vi "Process Packet.vi"(8 "error in (no error)":errorcluster, 10 "Incoming Packet":refnum<class "ControlPacket.lvclass">, 11 "Session in":refnum<class "Session.lvclass">) -> (0 "error out":errorcluster, 3 "Session out":refnum<class "Session.lvclass">)   [LabVIEW 2013, in "MQTT Base.lvlib" / "Session.lvclass"]
uses:
  Session.lvclass
  <vilib>/LabVIEW Open Source Project/MQTT Control Packets/Control Packets/ControlPacket/ControlPacket.lvclass
  Base Class/Request -- cluster.ctl
  Base Class/Response -- cluster.ctl
  Session.lvclass/Session.ctl
  <vilib>/LabVIEW Open Source Project/MQTT Control Packets/Control Packets/ControlPacket/ControlPacket.lvclass/ControlPacket.ctl
  Read SessionState.vi
  Base Class/MQTT_Base.lvclass
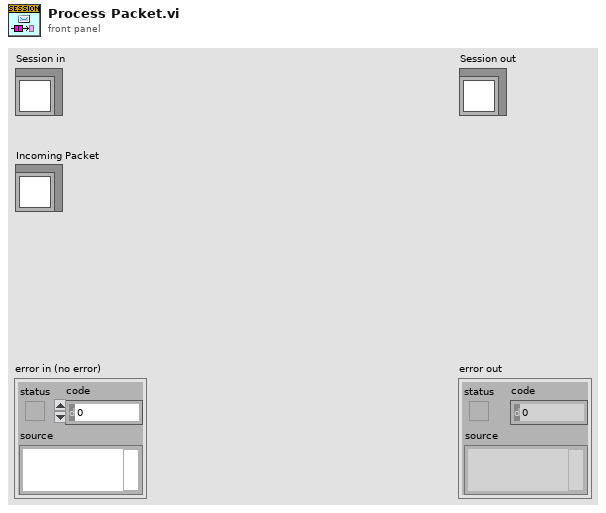
[diagram p1: front panel]
types:
  T1 = typedef "MQTT Base.lvlib/MQTT_Base.lvclass/Request -- cluster.ctl" = cluster{"Packet":refnum<class "ControlPacket.lvclass">, "SessionMailbox":refnum<queue>}
  T2 = typedef "MQTT Base.lvlib/MQTT_Base.lvclass/Response -- cluster.ctl" = cluster{"Packet":refnum<class "ControlPacket.lvclass">, "Protocol Error":errorcluster, "disconnect session":bool, "[ACK]":refnum<notifier>[]}
  T3 = typedef "MQTT Base.lvlib/Session.lvclass/Pending ACKs -- cluster.ctl" = cluster{"Message":refnum<class "ControlPacket.lvclass">, "[ACK]":refnum<notifier>[], "Packet Identifier":u16}
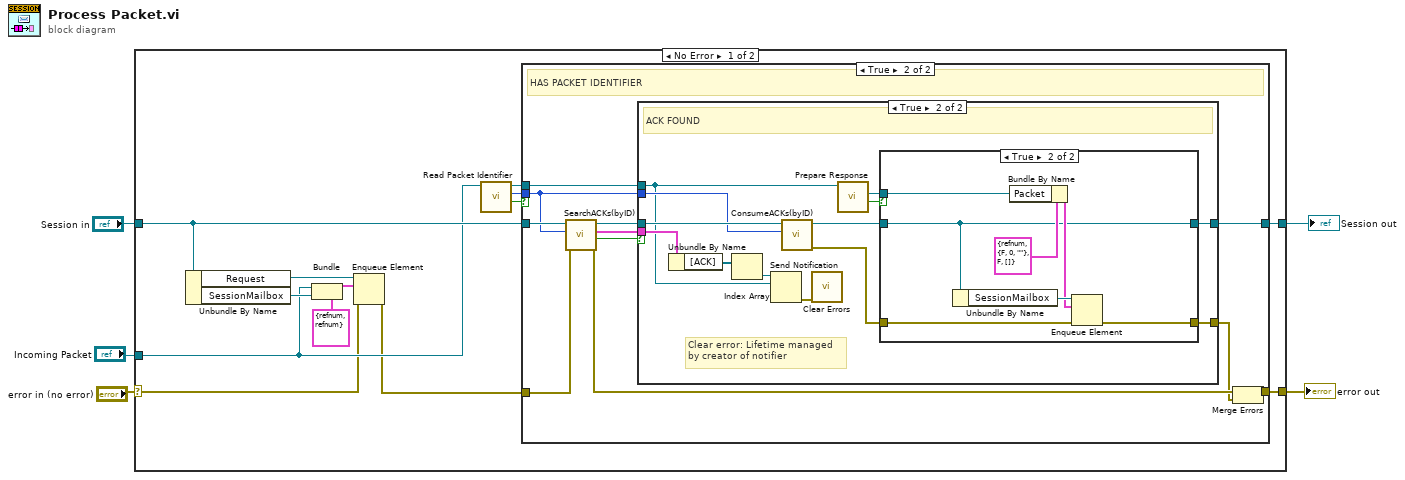
[diagram p0: block diagram]
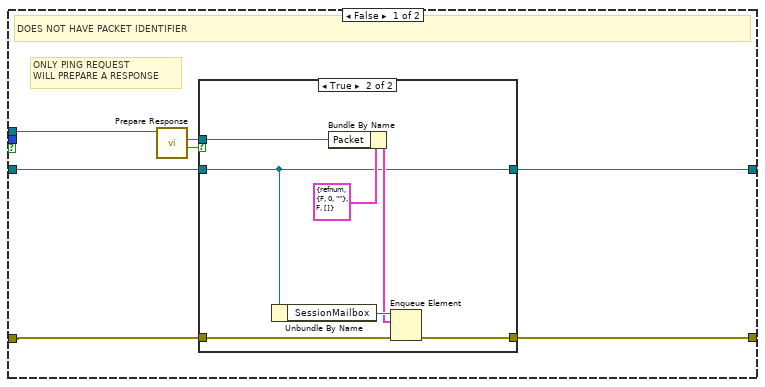
[diagram p2: hidden frame]
diagram:
  n1 = case shown="No Error" "error in (no error)" {
    selector: "error in (no error)" -> [w8 w70]
    tunnel: [w18 w70] -> w1
    tunnel: [w15 w69] -> w2
    tunnel: "Session in" -> [w10 w69]
    tunnel: "Incoming Packet" -> [w9 _]
    frame No Error {
      n2 = Unbundle By Name(w10) -> ("Request"=w11:refnum<queue>, "SessionMailbox"=w12:refnum<queue>)
      n3 = Bundle(cluster=T1 {"Packet"=refnum, "SessionMailbox"=refnum} ("Request"), "Packet"=w9, "SessionMailbox"=w12) -> (w13:T1)
      n4 = Enqueue Element(queue=w11, element=w13, error in (no error)=w8) -> (error out=w7:errorcluster)  [unwired: 1 in, 2 out]
      n5 = call <vilib>:"Read Packet Identifier.vi"("ControlPacket in"=w9) -> ("Has Packet Identifier"=w6:bool, "Packet Identifier"=w17:u16, "ControlPacket out"=w16:refnum<class "ControlPacket.lvclass">)  [unwired: 8 in]
      n6 = case shown="True" w6 {
        tunnel: [w19 w42] -> w18
        tunnel: w17 -> [_ w35]
        tunnel: w16 -> [w21 w41]
        tunnel: [w23 w39] -> w15
        tunnel: w10 -> [w24 w37]
        tunnel: w7 -> [w20 w36]
        frame False {
          # "ONLY PING REQUEST\nWILL PREPARE A RESPONSE"
          # "DOES NOT HAVE PACKET IDENTIFIER"
          n7 = call-dynamic "Prepare Response.vi"("ControlPacket in"=w21) -> ("response prepared?"=w22:bool, "ControlPacket response"=w25:refnum<class "ControlPacket.lvclass">)  [unwired: 7 in, 2 out]
          n8 = case shown="True" w22 {
            tunnel: w24 -> [w27 w29]
            tunnel: [w26 w31] -> w19
            tunnel: [w27 w29] -> w23
            tunnel: w25 -> [_ w30]
            tunnel: w20 -> [w26 w28]
            frame False {
            }
            frame True {
              n9 = Unbundle By Name(w29) -> ("SessionMailbox"=w34:refnum<queue>)
              n10 = Bundle By Name(cluster=T2 {"Packet"=refnum, "Protocol Error"={"status"=FALSE, "code"=0, "source"=""}, "disconnect session"=FALSE, "[ACK]"=[]} ("element"), "Packet"=w30) -> (w32:T2)
              n11 = Enqueue Element(queue=w34, element=w32, error in (no error)=w28) -> (error out=w31:errorcluster)  [unwired: 1 in, 2 out]
            }
          }
        }
        frame True {
          # "HAS PACKET IDENTIFIER"
          n12 = call "SearchACKs(byID).vi"("error in (no error)"=w36, "Packet Identifier"=w35, "Session in"=w37) -> ("error out"=w40:errorcluster, "found?"=w45:bool, "Pending ACK"=w44:T3, "Session out"=w43:refnum<class "Session.lvclass">)  [unwired: 5 in]
          n13 = case shown="True" w45 {
            tunnel: w44 -> [_ w56]
            tunnel: w43 -> [w46 w55]
            tunnel: [w46 w54] -> w39
            tunnel: w41 -> [_ w47]
            tunnel: [_ w53] -> w38
            tunnel: w35 -> [_ w48]
            frame False {
            }
            frame True {
              # "Clear error: Lifetime managed\nby creator of notifier"
              # "ACK FOUND"
              n14 = Unbundle By Name(w56) -> ("[ACK]"=w59:refnum<notifier>[])
              n15 = Index Array(array=w59) -> (element=w58:refnum<notifier>)  [unwired: 1 in]
              n16 = Send Notification(notification=w47, notifier=w58) -> (error out=w57:errorcluster)  [unwired: 1 in, 1 out]
              n17 = call "ConsumeACKs(byID).vi"("Packet Identifier"=w48, "Session in"=w55) -> ("error out"=w49:errorcluster, "Session out"=w50:refnum<class "Session.lvclass">)  [unwired: 8 in]
              n18 = call <vilib>:"Clear Errors.vi"("error in (no error)"=w57) -> ()  [unwired: 6 in, 1 out]
              n19 = call-dynamic "Prepare Response.vi"("ControlPacket in"=w47) -> ("response prepared?"=w52:bool, "ControlPacket response"=w51:refnum<class "ControlPacket.lvclass">)  [unwired: 7 in, 2 out]
              n20 = case shown="True" w52 {
                tunnel: w50 -> [w61 w62]
                tunnel: [w60 w65] -> w53
                tunnel: [w61 w62] -> w54
                tunnel: w51 -> [_ w64]
                tunnel: w49 -> [w60 w63]
                frame False {
                }
                frame True {
                  n21 = Unbundle By Name(w62) -> ("SessionMailbox"=w68:refnum<queue>)
                  n22 = Bundle By Name(cluster=T2 {"Packet"=refnum, "Protocol Error"={"status"=FALSE, "code"=0, "source"=""}, "disconnect session"=FALSE, "[ACK]"=[]} ("element"), "Packet"=w64) -> (w66:T2)
                  n23 = Enqueue Element(queue=w68, element=w66, error in (no error)=w63) -> (error out=w65:errorcluster)  [unwired: 1 in, 2 out]
                }
              }
            }
          }
          n24 = Merge Errors(w40, w38) -> (w42:errorcluster)
        }
      }
    }
    frame Error {
    }
  }
  "error out" <- w1
  "Session out" <- w2
